vi "Change Theme.vi"(8 "error in (no error)":errorcluster, 10 "Filled Text Fields.Theme":T1={"Main"={"Primary"=15224622, "Primary Variant"=16744512, "Secondary"=9342606, "Secondary Varient"=2039583}, "Container"={"BG"=16119285, "Hover"=15527148, "Focused"=14474460}, "Text"={"Default"=5855577, "Error"=11534368}}, 11 "Filled Text Fields Actor in":refnum<class "Filled Text Fields Actor.lvclass">) -> (0 "error out":errorcluster, 3 "Filled Text Fields Actor out":refnum<class "Filled Text Fields Actor.lvclass">)   [LabVIEW 2017, in "Filled Text Fields Actor.lvlib" / "Filled Text Fields Actor.lvclass"]
uses:
  Filled Text Fields Actor.lvclass
  Filled Text Fields.Theme.Colors.ctl
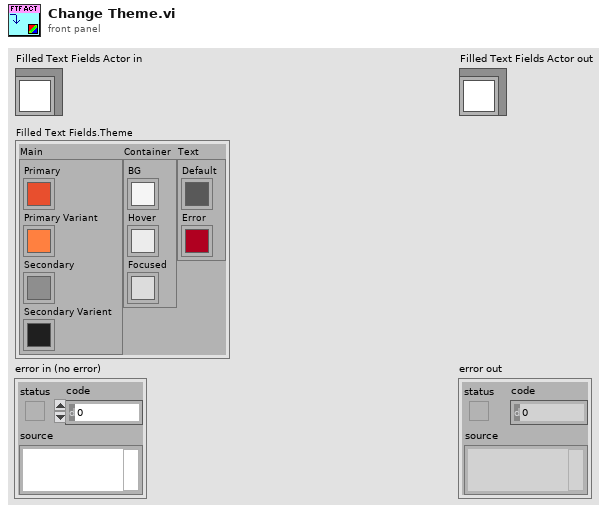
[diagram p1: front panel]
types:
  T1 = typedef "Filled Text Fields Actor.lvlib/Filled Text Fields Actor.lvclass/Filled Text Fields.Theme.Colors.ctl" = cluster{"Main":cluster{"Primary":u32, "Primary Variant":u32, "Secondary":u32, "Secondary Varient":u32}, "Container":cluster{"BG":u32, "Hover":u32, "Focused":u32}, "Text":cluster{"Default":u32, "Error":u32}}
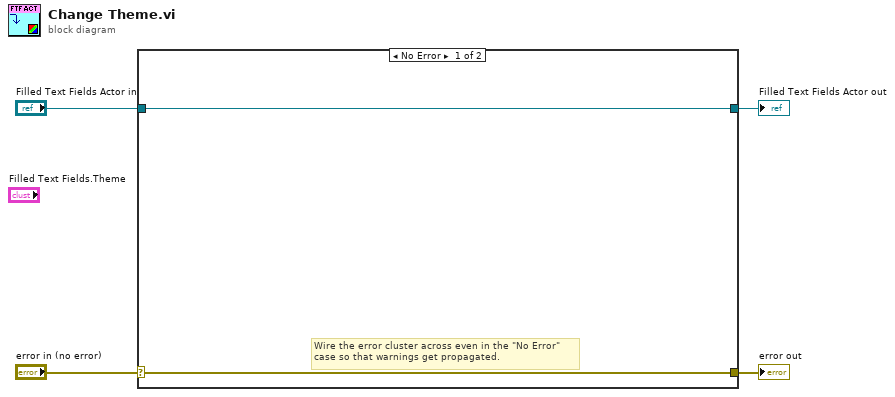
[diagram p0: block diagram]
diagram:
  n1 = case shown="No Error" "error in (no error)" {
    selector: "error in (no error)" -> [w5 w8]
    tunnel: [w5 w8] -> w3
    tunnel: [w6 w7] -> w1
    tunnel: "Filled Text Fields Actor in" -> [w6 w7]
    frame No Error {
      # "Wire the error cluster across even in the \"No Error\"\ncase so that warnings get propagated."
    }
    frame Error {
    }
  }
  "error out" <- w3
  "Filled Text Fields Actor out" <- w1
